vi "Hahn Echo with Pi Pulse Contrast.vi"() -> ()   [LabVIEW 2012]
uses:
  <vilib>/DAQmx/read.llb/DAQmx Read (Counter U32 1Chan 1Samp).vi
  <vilib>/Utility/file.llb/Write To Spreadsheet File (DBL).vi
  <vilib>/DAQmx/create/channels.llb/DAQmx Create Channel (CI-Count Edges).vi
  <vilib>/DAQmx/configure/timing.llb/DAQmx Timing (Sample Clock).vi
  <vilib>/DAQmx/create/channels.llb/DAQmx Create Channel (CO-Pulse Generation-Ticks).vi
  <vilib>/DAQmx/configure/timing.llb/DAQmx Timing (Implicit).vi
  <vilib>/Utility/file.llb/Write To Spreadsheet File (I64).vi
  <vilib>/DAQmx/miscellaneous.llb/DAQmx Fill In Error Info.vi
  <resource>/objmgr/daqmx.rc
panel:
  out "Tracking loop":i32=37
  in  "Z-track?":bool=TRUE
  in  "Z Pos":dbl=50.8
  in  "Y pos":dbl=100.0
  in  "X Pos":dbl=40.0
  in  "Total time":i32=3600
  in  "Tracking Interval":dbl=150.0
  in  "stop":bool
  out "pi":u32=52
  out "no pi":u32=53
  in  "Path to spinapi.dll":path=path "C:/SpinCore/SpinAPI/dll/spinapi64.dll"
  in  "file path (dialog if empty)":path
  in  "AOM Rest time":dbl=1e-06
  in  "Rabi Freq":dbl=8640000.0
  in  "MW Delay":dbl=5e-08
  in  "type":u16(ring) items=["Linear", "Logarithmic"]
  in  "Tau No. Steps":i32=40
  in  "Tau Min":dbl=2e-08
  in  "Tau Max":dbl=1e-06
  in  "Signal Delay":dbl=7.6e-07
  in  "APD signal width":dbl=3e-07
  in  "AOM Pulse length":dbl=2.5e-06
  in  "N Loop":i32=100000
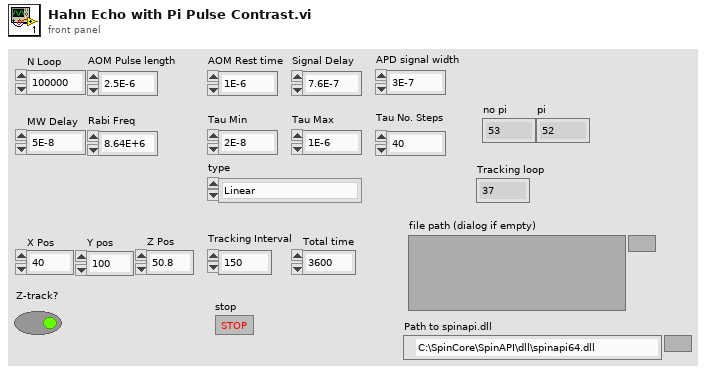
[diagram p1: front panel]
types:
  T1 = cluster{"Number of Y Steps":i32, "Max Y (V)":dbl, "Min Y (V)":dbl}
  T2 = cluster{"Number of X Steps":i32, "Max X (V)":dbl, "Min X (V)":dbl}
  T3 = cluster{"Instruct Data":i32, "Op Code":i32, "Flags":bool[], "Comments":string, "Time (s)":dbl}
  T4 = enum16{"Pulse Program", "Frequency Registers", "TX Phase Registers", "RX Phase Registers"}
  T5 = cluster{"Instruct Data":i32, "Op Code":i32, "Flags":bool[], "Comments":string, "Time (s)":dbl}[]
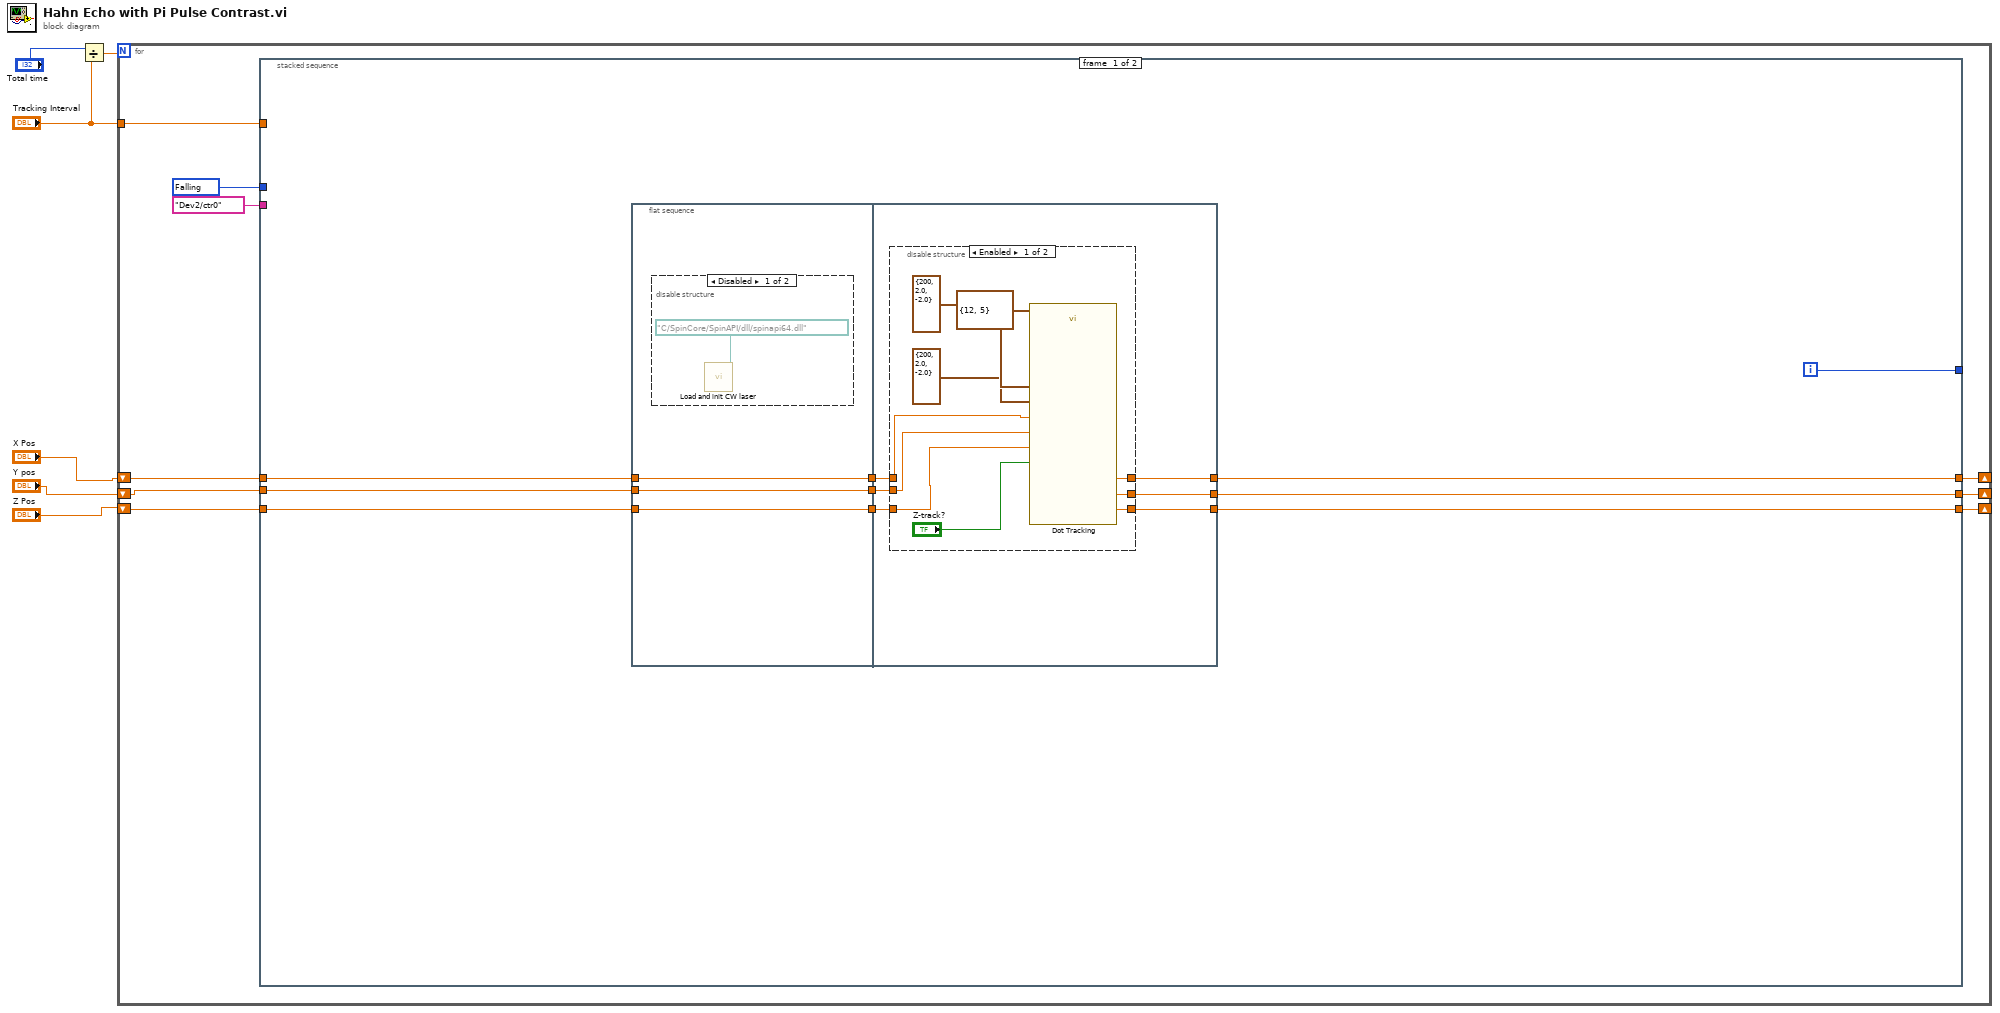
[diagram p0: block diagram]
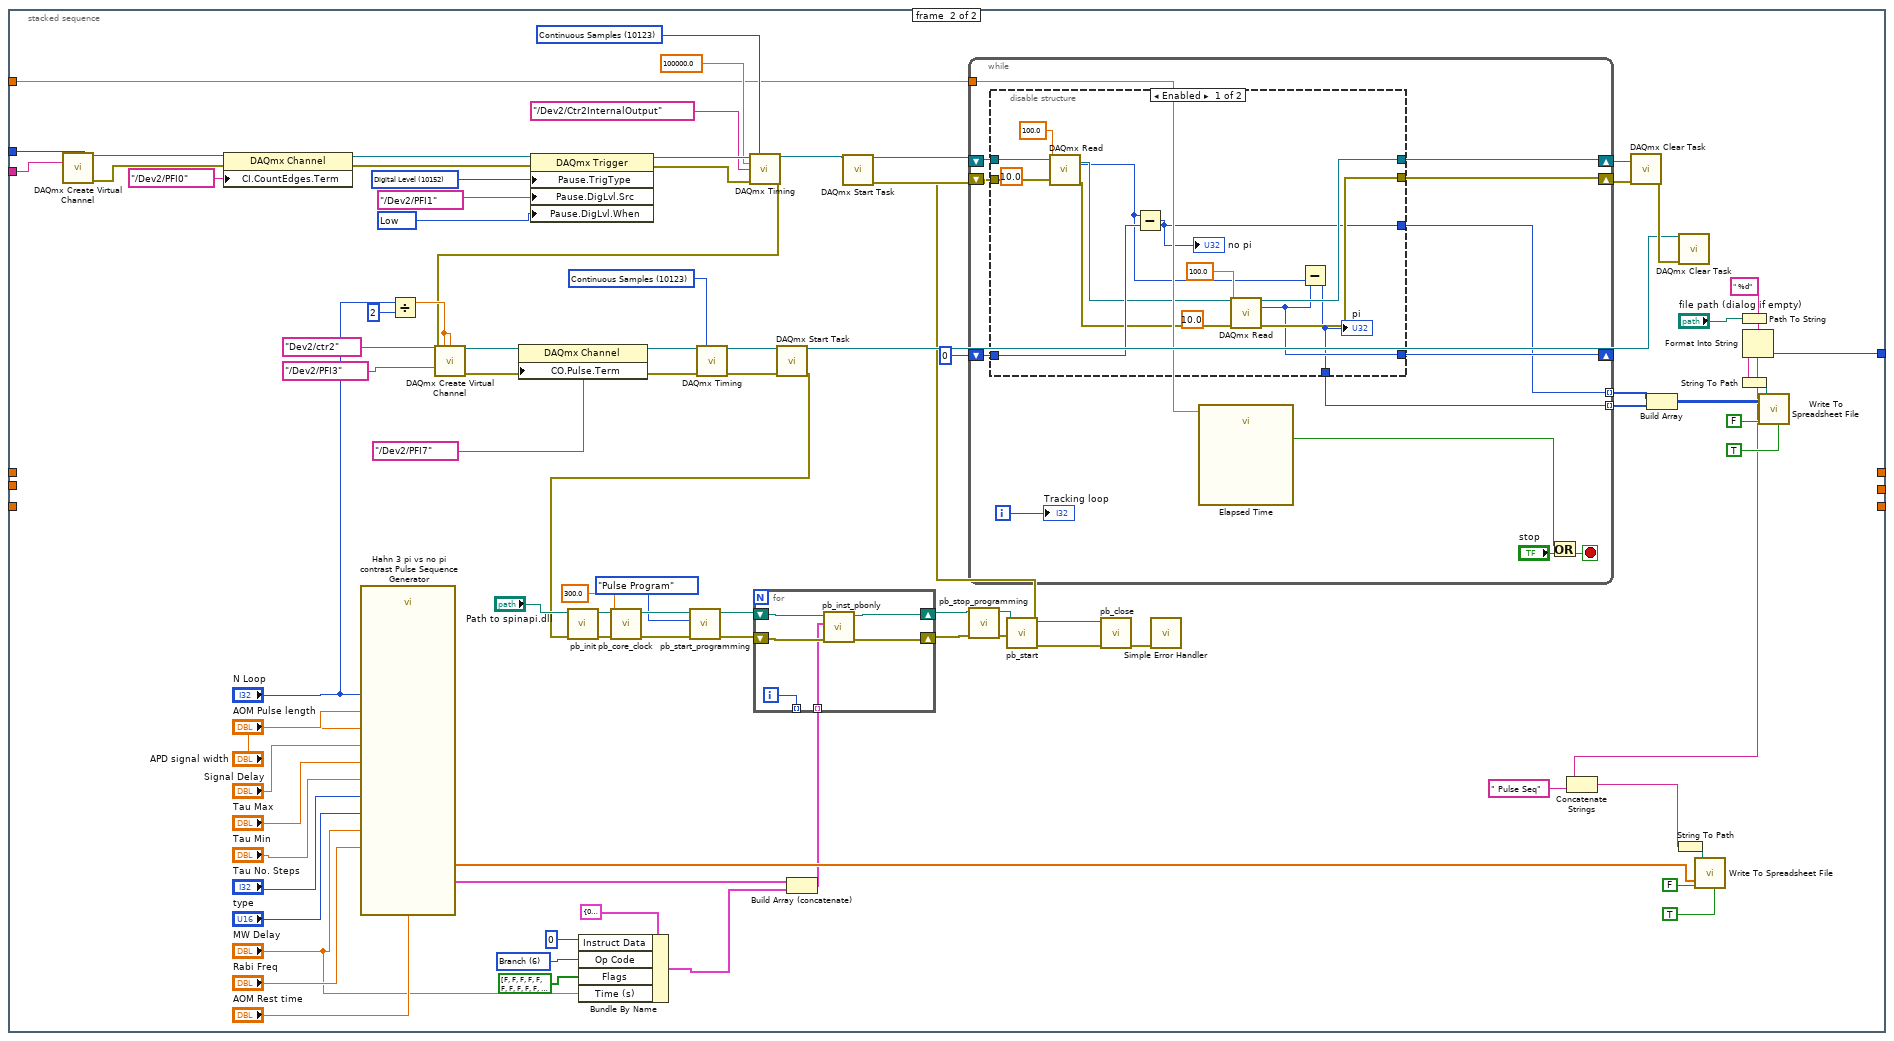
[diagram p4: hidden frame]
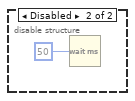
[diagram p5: hidden frame]
diagram:
  n1 = Divide(x="Total time", y="Tracking Interval") -> (x/y=w3:dbl)
  n2 = for {
    N: w3 -> [_]
    shift-right: [w13] -> _
    shift-left: "X Pos" -> [w10]
    shift-right: [w12] -> _
    shift-left: "Y pos" -> [w9]
    shift-right: [w11] -> _
    shift-left: "Z Pos" -> [w8]
    tunnel: "Tracking Interval" -> [w7]
    i -> [w14]
    w15 = 10171 items=["Rising"=10280, "Falling"=10171] ("edge")
    n3 = stacked-sequence {
      tunnel: tag "Dev2/ctr0" ("counter") -> [_ w124]
      tunnel: w15 -> [_ w123]
      tunnel: w14 -> [_ w66]
      tunnel: [w25 _] -> w13
      tunnel: [w24 _] -> w12
      tunnel: [w23 _] -> w11
      tunnel: w10 -> [w21 _]
      tunnel: w9 -> [w20 _]
      tunnel: w8 -> [w17 _]
      tunnel: w7 -> [_ w62]
      frame #0 {
        n4 = flat-sequence {
          tunnel: [w28] -> w22
          tunnel: w21 -> [w28]
          tunnel: w20 -> [w27]
          tunnel: [w27] -> w19
          tunnel: [w26] -> w18
          tunnel: w17 -> [w26]
          tunnel: [w35] -> w25
          tunnel: [w34] -> w24
          tunnel: [w33] -> w23
          tunnel: w22 -> [w32]
          tunnel: w19 -> [w31]
          tunnel: w18 -> [w30]
          frame #0 {
            n5 = disable-structure shown="Disabled" {
              frame Disabled {
                n6 = call "Load and init CW laser.vi"("path in"=path "C:/SpinCore/SpinAPI/dll/spinapi64.dll") -> ()  [unwired: 11 in]
              }
              frame Enabled {
              }
            }
          }
          frame #1 {
            n7 = disable-structure shown="Enabled" {
              disable-tunnel: [w41 _] -> w35
              disable-tunnel: [w40 _] -> w34
              disable-tunnel: [w39 _] -> w33
              disable-tunnel: w32 -> [w38 _]
              disable-tunnel: w31 -> [w37 _]
              disable-tunnel: w30 -> [w36 _]
              frame Enabled {
                n8 = call "Dot Tracking.vi"("X"=T2 {"Number of X Steps"=200, "Max X (V)"=2.0, "Min X (V)"=-2.0}, "Y Parameters"=T1 {"Number of Y Steps"=200, "Max Y (V)"=2.0, "Min Y (V)"=-2.0}, "RS232 settings"=cluster{"Portnumber":i32, "Baudrate":u16} {"Portnumber"=12, "Baudrate"=5}, "X Pos"=w38, "Y pos"=w37, "Z Pos"=w36, "Z-track?"="Z-track?") -> ("X Position"=w41:dbl, "Y Position"=w40:dbl, "Z Position"=w39:dbl)  [unwired: 2 in, 4 out]
              }
              frame Disabled {
              }
            }
          }
        }
      }
      frame #1 {
        w52 = 6 items=["Continue", "Stop", "Loop", "End Loop", "JSR", "RTS", "Branch", "Long Delay", "Wait"] ("Op Code")
        w100 = 10123 items=["Finite Samples"=10178, "Continuous Samples"=10123, "Hardware Timed Single Point"=12522] ("sample mode")
        w120 = 10214 items=["High"=10192, "Low"=10214] ("Pause.DigLvl.When")
        w122 = 10152 items=["Analog Level"=10101, "Analog Window"=10103, "Digital Level"=10152, "Digital Pattern"=10398, "None"=10230] ("Pause.TrigType")
        w109 = 10123 items=["Finite Samples"=10178, "Continuous Samples"=10123, "Hardware Timed Single Point"=12522] ("sample mode")
        n9 = call-poly <vilib>:"DAQmx Create Virtual Channel.vi"("edge"=w123, "counter"=w124) -> ("task out"=w118:refnum<k21>, "error out"=w115:errorcluster)  [unwired: 7 in, 5 out]
        n10 = property class="DAQmx Channel"(reference=w118, error in=w115, "CI.CountEdges.Term"=tag "/Dev2/PFI0") -> (reference out=w119:refnum<k21>, error out=w117:errorcluster)
        n11 = call "Hahn 3 pi vs no pi contrast Pulse Sequence Generator.vi"("N Loop"="N Loop", "Rabi Freq"="Rabi Freq", "Tau Min"="Tau Min", "AOM Pulse length"="AOM Pulse length", "AOM Rest time"="AOM Rest time", "Signal Delay"="Signal Delay", "Tau No. Steps"="Tau No. Steps", "APD signal width"="APD signal width", "MW Delay"="MW Delay", "Tau Max"="Tau Max", "type"="type") -> ("Pulse Sequence"=w75:T5, "Tau"=w58:dbl[])  [unwired: 3 in]
        n12 = Divide(x="N Loop", y=2) -> (x/y=w106:dbl)
        n13 = property class="DAQmx Trigger"(reference=w119, error in=w117, "Pause.TrigType"=w122, "Pause.DigLvl.Src"=tag "/Dev2/PFI1", "Pause.DigLvl.When"=w120) -> (reference out=w114:refnum<k21>, error out=w113:errorcluster)
        n14 = Bundle By Name(cluster=T3 {"Instruct Data"=0, "Op Code"=0, "Flags"=[FALSE, FALSE, FALSE, FALSE, FALSE, FALSE, FALSE, FALSE, FALSE, FALSE, FALSE, FALSE, FALSE, FALSE, FALSE, FALSE, FALSE, FALSE, FALSE, FALSE, FALSE, TRUE, TRUE, TRUE], "Comments"="", "Time (s)"=0.01} ("PB Inst 2"), "Instruct Data"=0, "Op Code"=w52, "Flags"=bool[] [FALSE, FALSE, FALSE, FALSE, FALSE, FALSE, FALSE, FALSE, FALSE, FALSE, FALSE, FALSE, FALSE, FALSE, FALSE, FALSE, FALSE, FALSE, FALSE, FALSE, FALSE, TRUE, TRUE, TRUE], "Time (s)"="MW Delay") -> (w49:T3)
        n15 = call-poly <vilib>:"DAQmx Timing.vi"("task/channels in"=w114, "sample mode"=w109, "rate"=100000.0, "source"=tag "/Dev2/Ctr2InternalOutput", "error in"=w113) -> ("task out"=w111:refnum<k21>, "error out"=w46:errorcluster)  [unwired: 9 in]
        n16 = call-poly <vilib>:"DAQmx Create Virtual Channel.vi"("high ticks"=w106, "low ticks"=w106, "counter"=tag "Dev2/ctr2", "source of ticks"=tag "/Dev2/PFI3" ("source"), "error in"=w46) -> ("task out"=w104:refnum<k21>, "error out"=w102:errorcluster)  [unwired: 9 in]
        n17 = property class="DAQmx Channel"(reference=w104, "CO.Pulse.Term"=tag "/Dev2/PFI7") -> (reference out=w99:refnum<k21>)  [unwired: 1 in, 1 out]
        n18 = call-poly <vilib>:"DAQmx Timing.vi"("task/channels in"=w99, "sample mode"=w100, "error in"=w102) -> ("task out"=w103:refnum<k21>, "error out"=w101:errorcluster)  [unwired: 11 in]
        n19 = call <vilib>:"DAQmx Start Task.vi"("task/channels in"=w103, "error in"=w101) -> ("task out"=w91:refnum<k21>, "error out"=w76:errorcluster)  [unwired: 12 in]
        n20 = call "pb_init.vi"("error in (no error)"=w76, "path in"="Path to spinapi.dll") -> ("error out"=w80:errorcluster, "path out"=w78:path)  [unwired: 2 in, 6 out]
        n21 = call "pb_core_clock.vi"("error in (no error)"=w80, "clock_freq (MHz)"=300.0, "path in"=w78) -> ("error out"=w81:errorcluster, "path out"=w79:path)  [unwired: 7 in]
        n22 = call "pb_start_programming.vi"("error in (no error)"=w81, "Device"=T4."Pulse Program", "path in"=w79) -> ("error out"=w84:errorcluster, "path out"=w83:path)  [unwired: 1 in, 6 out]
        n23 = Build Array (concatenate)(w75, w49) -> (w50:T5)
        n24 = for {
          shift-right: [w164] -> w85
          shift-left: w83 -> [w166]
          shift-right: [w163] -> w86
          shift-left: w84 -> [w165]
          tunnel: [w162] -> _ mode=indexing
          tunnel: w50 -> [w161] mode=indexing
          i -> [w162]
          n25 = call "pb_inst_pbonly.vi"("error in (no error)"=w165, "PB Instruction"=w161, "path in"=w166) -> ("error out"=w163:errorcluster, "path out"=w164:path)  [unwired: 2 in, 5 out]
        }
        n26 = call "pb_stop_programming.vi"("error in (no error)"=w86, "path in"=w85) -> ("error out"=w73:errorcluster, "path out"=w74:path)  [unwired: 1 in, 7 out]
        n27 = call "pb_start.vi"("error in (no error)"=w73, "path in"=w74) -> ("error out"=w47:errorcluster, "path out"=w72:path)  [unwired: 1 in, 7 out]
        n28 = call <vilib>:"DAQmx Start Task.vi"("task/channels in"=w111, "error in"=w47) -> ("task out"=w95:refnum<k21>, "error out"=w94:errorcluster)  [unwired: 12 out]
        n29 = while {
          shift-right: [w142] -> w96
          shift-left: w95 -> [w146]
          shift-right: [w141] -> _
          shift-left: u32 0 ("data") -> [w145]
          shift-right: [w143] -> w93
          shift-left: w94 -> [w144]
          tunnel: [w137] -> w70 mode=indexing
          tunnel: [w136] -> w69 mode=indexing
          tunnel: w62 -> [w135]
          i -> [w134]
          stop <- w139 stop-if-true
          n30 = disable-structure shown="Enabled" {
            disable-tunnel: w146 -> [w159 _]
            disable-tunnel: w145 -> [w158 _]
            disable-tunnel: w144 -> [w157 _]
            disable-tunnel: [w151 _] -> w143
            disable-tunnel: [w150 _] -> w142
            disable-tunnel: [w149 _] -> w141
            disable-tunnel: [w148 _] -> w137
            disable-tunnel: [w147 _] -> w136
            frame Enabled {
              (unwired) 10.0 ("timeout")
              (unwired) 10.0 ("timeout")
              n31 = call-poly <vilib>:"DAQmx Read.vi"("task/channels in"=w159, "timeout"=100.0, "error in"=w157) -> ("task out"=w155:refnum<k21>, "data"=w152:u32, "error out"=w154:errorcluster)  [unwired: 10 in]
              n32 = Subtract(x=w152, y=w158) -> (x-y=w148:u32)
              "no pi" <- w148
              n33 = call-poly <vilib>:"DAQmx Read.vi"("task/channels in"=w155, "timeout"=100.0, "error in"=w154) -> ("task out"=w150:refnum<k21>, "data"=w149:u32, "error out"=w151:errorcluster)  [unwired: 10 in]
              n34 = Subtract(x=w149, y=w152) -> (x-y=w147:u32)
              "pi" <- w147
            }
            frame Disabled {
              n35 = Wait (ms)(milliseconds to wait=u32 50) -> ()  [unwired: 1 out]
            }
          }
          n36 = call "Elapsed Time"("Time Target (s)"=w135) -> ("Time has Elapsed"=w138:bool)  [unwired: 11 in, 7 out]
          n37 = Or(x=w138, y="stop") -> (x .or. y?=w139:bool)
          "Tracking loop" <- w134
        }
        n38 = call "pb_close.vi"("error in (no error)"=w47, "path in"=w72) -> ("error out"=w88:errorcluster)  [unwired: 9 out]
        n39 = call <vilib>:"Simple Error Handler.vi"("error in (no error)"=w88) -> ()  [unwired: 1 in, 8 out]
        n40 = call <vilib>:"DAQmx Clear Task.vi"("task in"=w96, "error in"=w93) -> ("error out"=w92:errorcluster)  [unwired: 13 in]
        n41 = Build Array(w70, w69) -> (w68:u32[][])
        n42 = call <vilib>:"DAQmx Clear Task.vi"("task in"=w91, "error in"=w92) -> ()  [unwired: 13 in, 1 out]
        n43 = Path To String(path="file path (dialog if empty)") -> (string=w57:string)
        n44 = Concatenate Strings(w57, " Pulse Seq" ("string")) -> (w56:string)
        n45 = String To Path(string=w56) -> (path=w59:path)
        n46 = call-poly <vilib>:"Write To Spreadsheet File.vi"("transpose? (no:F)"=TRUE, "append to file? (new file:F)"=FALSE, "1D data"=w58, "file path (dialog if empty)"=w59) -> ()  [unwired: 4 in, 1 out]
        n47 = Format Into String(format string=" %d", initial string=w57, w66) -> (resulting string=w64:string)  [unwired: 1 in, 1 out]
        n48 = String To Path(string=w64) -> (path=w63:path)
        n49 = call-poly <vilib>:"Write To Spreadsheet File.vi"("transpose? (no:F)"=TRUE, "append to file? (new file:F)"=FALSE, "2D data"=w68, "file path (dialog if empty)"=w63) -> ()  [unwired: 4 in, 1 out]
      }
    }
  }
